vi "scaleSqWaveParams.vi"(0 "clock rate (Hz)":dbl=40000000.0 format="%#_6p", 5 "max voltage for target":dbl=10.0, 7 "square wave props":T2={"frequency (Hz)"=10000.0, "phase offset (deg)"=0.0, "amplitude (V peak)"=10.0, "offset (V)"=0.0, "duty cycle (%)"=50.0} {"frequency (Hz)" format="%#_6p"}, 11 "error in (no error)":errorcluster) -> (8 "scaled square wave props":T1 {"frequency (periods/tick)" format="%.32g"; "phase offset (periods)" format="%.32g"; "duty cycle (periods)" format="%.32g"}, 15 "error out":errorcluster)   [LabVIEW 2012]
uses:
  <vilib>/rvi/Analysis/host/Public/NI_FpgaMspHost.lvlib
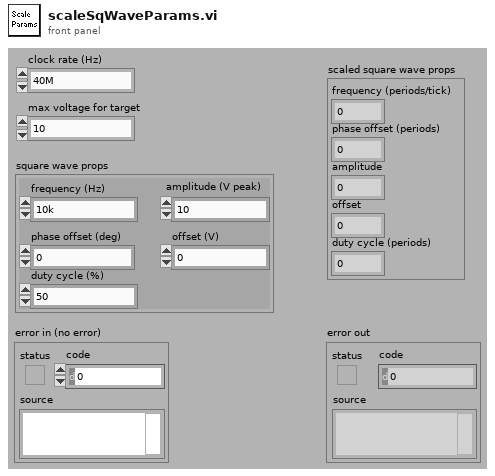
[diagram p1: front panel]
types:
  T1 = cluster{"frequency (periods/tick)":fxp<+,32,0>, "phase offset (periods)":fxp<+,32,0>, "amplitude":i16, "offset":i16, "duty cycle (periods)":fxp<+,32,0>}
  T2 = cluster{"frequency (Hz)":dbl, "phase offset (deg)":dbl, "amplitude (V peak)":dbl, "offset (V)":dbl, "duty cycle (%)":dbl}
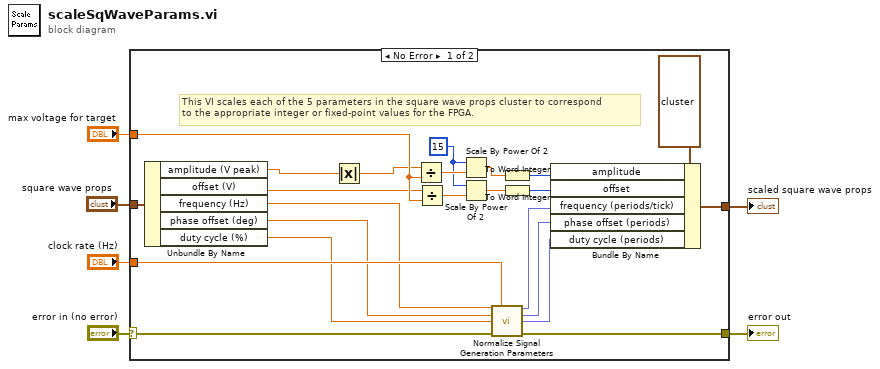
[diagram p0: block diagram]
diagram:
  n1 = case shown="No Error" "error in (no error)" {
    selector: "error in (no error)" -> [w20 w30]
    tunnel: [w29 _] -> w6
    tunnel: "square wave props" -> [w23 _]
    tunnel: "clock rate (Hz)" -> [w19 _]
    tunnel: "max voltage for target" -> [w22 _]
    tunnel: [w16 w30] -> w1
    frame No Error {
      w26 = 15 ("n")
      # "This VI scales each of the 5 parameters in the square wave props cluster to correspond\nto the appropriate integer or fixed-point values for the FPGA."
      n2 = Unbundle By Name(w23) -> ("amplitude (V peak)"=w11:dbl, "offset (V)"=w12:dbl, "frequency (Hz)"=w7:dbl, "phase offset (deg)"=w18:dbl, "duty cycle (%)"=w17:dbl)
      n3 = Absolute Value(x=w11) -> (abs(x)=w8:dbl)
      n4 = Divide(x=w8, y=w22) -> (x/y=w28:dbl)
      n5 = Divide(x=w12, y=w22) -> (x/y=w27:dbl)
      n6 = Scale By Power Of 2(n=w26, x=w28) -> (x*2^n=w25:dbl)
      n7 = Scale By Power Of 2(n=w26, x=w27) -> (x*2^n=w24:dbl)
      n8 = call <vilib>:"Normalize Signal Generation Parameters.vi"("frequency (Hz)"=w7, "FPGA clock rate (Hz)"=w19, "phase offset (deg)"=w18, "duty cycle (%)"=w17, "error in (no error)"=w20) -> ("frequency (periods/tick)"=w15:fxp<+,32,0>, "phase offset (periods)"=w14:fxp<+,32,0>, "duty cycle (periods)"=w13:fxp<+,32,0>, "error out"=w16:errorcluster)  [unwired: 5 in, 2 out]
      n9 = To Word Integer(number=w25) -> (16bit integer=w10:i16)
      n10 = To Word Integer(number=w24) -> (16bit integer=w9:i16)
      n11 = Bundle By Name(cluster=T1 {"frequency (periods/tick)"=0.9999999997671694, "phase offset (periods)"=0.0, "amplitude"=32767, "offset"=0, "duty cycle (periods)"=0.9999999997671694} ("Square wave 3"), "amplitude"=w10, "offset"=w9, "frequency (periods/tick)"=w15, "phase offset (periods)"=w14, "duty cycle (periods)"=w13) -> (w29:T1)
    }
    frame Error {
    }
  }
  "scaled square wave props" <- w6
  "error out" <- w1
